vi "rad_Deploy Image Wrapper_FB.vi"(4 "Deploy":string[](array[string]), 6 "restart after imaging (T)":bool=TRUE, 7 "Deployment Notifiers":T3, 8 "error in (no error)":errorcluster, 9 "apply primary NIC from image (F)":bool, 10 "image file path":path, 11 "Target settings in":T1={"Hostname"="", "Serial number"="", "Product name"="", "Product code"=0, "System status"="", "Credential type"=enum."None/Unlocked", "User added?"=FALSE, "Primary NIC"={"MAC address"="", "IP Address Request Mode"=2, "IP address"="", "Subnet mask"="", "Gateway"="", "DNS server"=""}} {"Primary NIC"."IP Address Request Mode" items=["Static"=1, "DHCP/Link-Local"=2, "Link-Local Only"=4, "DHCP Only"=8]}) -> (0 "error out":errorcluster, 2 "image file path":path, 3 "Target settings out":T1={"Hostname"="", "Serial number"="", "Product name"="", "Product code"=0, "System status"="", "Credential type"=enum."None/Unlocked", "User added?"=FALSE, "Primary NIC"={"MAC address"="", "IP Address Request Mode"=2, "IP address"="", "Subnet mask"="", "Gateway"="", "DNS server"=""}} {"Primary NIC"."IP Address Request Mode" items=["Static"=1, "DHCP/Link-Local"=2, "Link-Local Only"=4, "DHCP Only"=8]})   [LabVIEW 2014]
uses:
  TypeDefs/rad_Deployment Notifiers.ctl
  TypeDefs/rad_Deployment Status Data Type.ctl
  TypeDefs/rad_Deployment Progress Data Type.ctl
  Targets/TypeDefs/rad_Target Information.ctl
  Targets/TypeDefs/rad_Target Network Settings.ctl
  <vilib>/nisyscfg/Network Settings Image.ctl
  <vilib>/nisyscfg/Set System Image (Folder).vi
  <vilib>/nisyscfg/Set System Image (File).vi
  <vilib>/nisyscfg/Close (System).vi
  <vilib>/nisyscfg/nisyscfg.lvlib
panel:
  out "finished":bool
  in  "Stop Checking for Events":bool
  out "Progress":u8(slide) scale=0.0..100.0
  out "Status":string
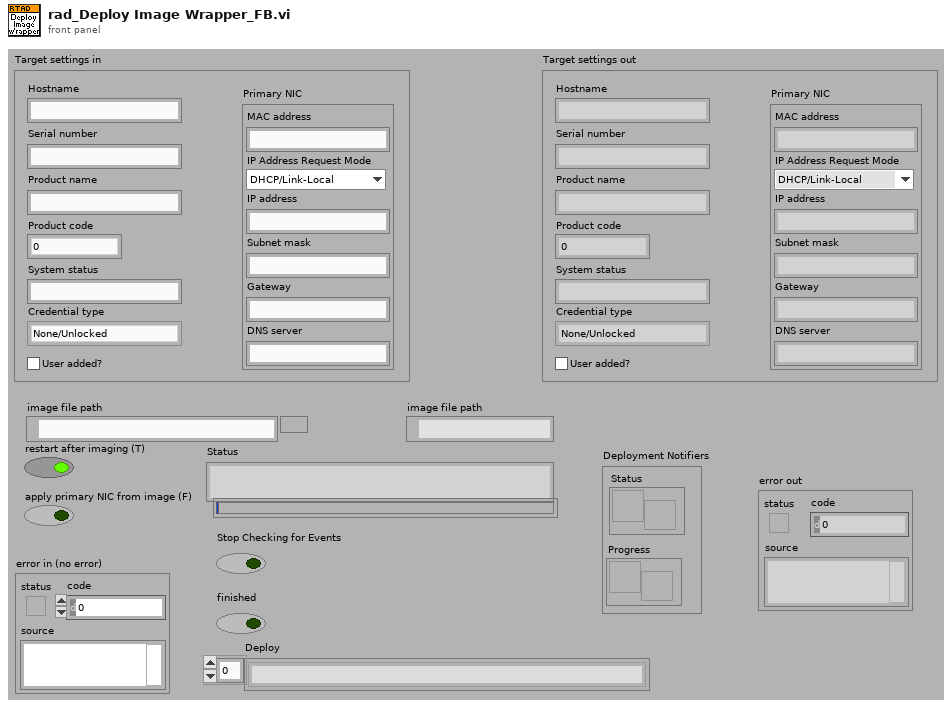
[diagram p1: front panel]
types:
  T1 = typedef "rad_Target Information.ctl" = cluster{"Hostname":string, "Serial number":string, "Product name":string, "Product code":i32, "System status":string, "Credential type":enum16{"None/Unlocked", "FTP Password", "NIAuth Credentials"}, "User added?":bool, "Primary NIC":T2}
  T2 = typedef "rad_Target Network Settings.ctl" = cluster{"MAC address":string, "IP Address Request Mode":i32, "IP address":string, "Subnet mask":string, "Gateway":string, "DNS server":string}
  T3 = typedef "rad_Deployment Notifiers.ctl" = cluster{"Status":refnum<notifier>, "Progress":refnum<notifier>}
  T4 = typedef "rad_Deployment Progress Data Type.ctl" = i8
  T5 = typedef "nisyscfg.lvlib/Network Settings Image.ctl" = u32
  T6 = enum32{"state changed", "beginning restart", "getting file", "putting file", "creating directory", "deleting file", "deleting directory", "enumerating file system", "renaming file", "current component", "operation progress", "downloading file", "unpacking file", "running install script"}
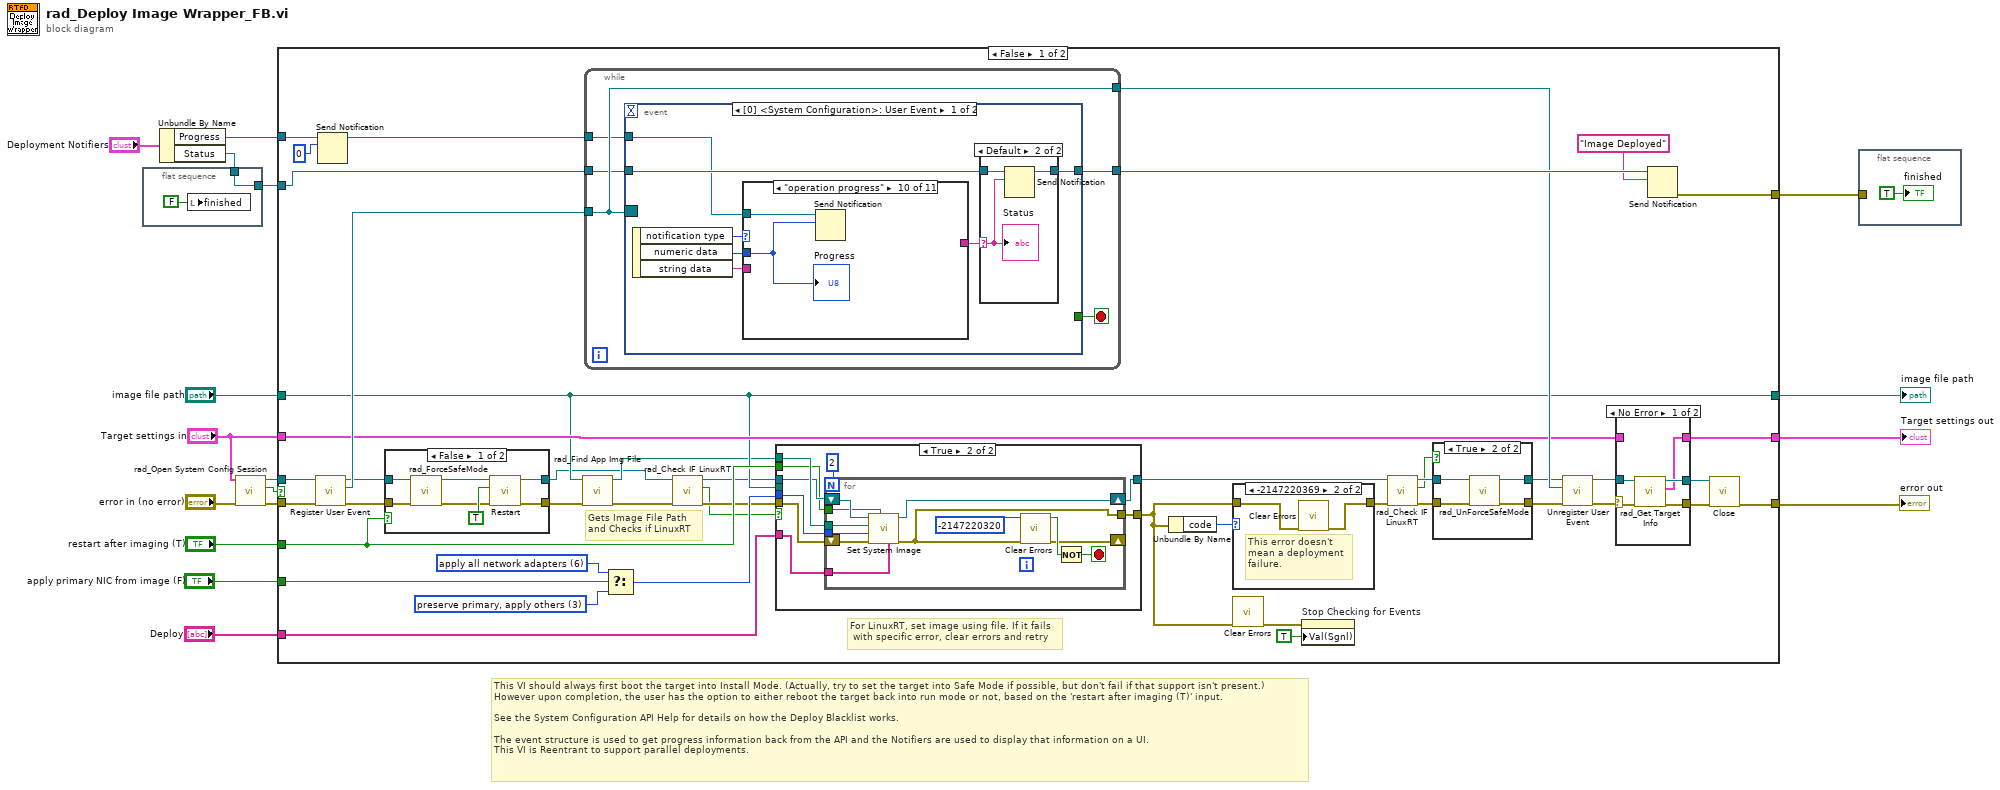
[diagram p0: block diagram]
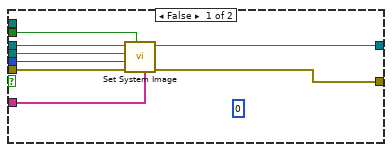
[diagram p2: hidden frame]
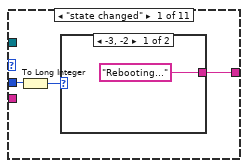
[diagram p8: hidden frame]
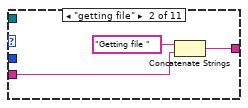
[diagram p10: hidden frame]
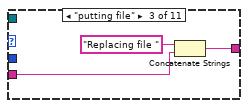
[diagram p11: hidden frame]
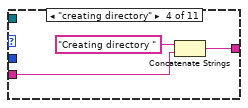
[diagram p12: hidden frame]
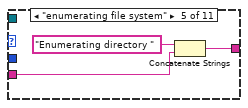
[diagram p13: hidden frame]
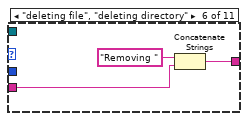
[diagram p14: hidden frame]
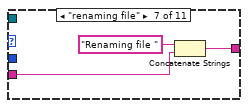
[diagram p15: hidden frame]
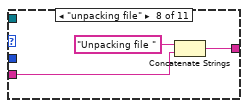
[diagram p16: hidden frame]
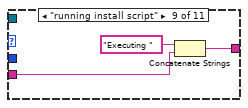
[diagram p17: hidden frame]
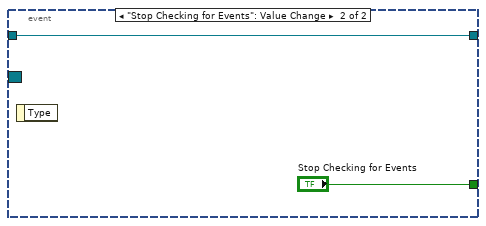
[diagram p19: hidden frame]
diagram:
  # "This VI should always first boot the target into Install Mode. (Actually, try to set the target into Safe Mode if possible, but don't fail if that support isn't present.)\nHowever upon completion, the user has the option to either reboot the target back into run mode or not, based on the 'restart after imaging (T)' input.\n\nSee the System Configuration API Help for details on how the Deploy Blacklist works.\n\nThe event structure is used to get progress information back from the API and the Notifiers are used to display that information on a UI. \nThis VI is Reentrant to support parallel deployments."
  n1 = flat-sequence {
    tunnel: [w18] -> w3
    tunnel: w2 -> [w18]
    frame #0 {
      n2 = local write "finished"(FALSE ("finished")) -> ()
    }
  }
  n3 = Unbundle By Name("Deployment Notifiers") -> ("Progress"=w11:refnum<notifier>, "Status"=w2:refnum<notifier>)
  n4 = call "rad_Open System Config Session.vi"("error in (no error)"="error in (no error)", "Target settings"="Target settings in") -> ("error out"=w7:errorcluster, "Cancelled"=w6:bool, "Session out"=w8:refnum<k21>)  [unwired: 6 in, 1 out]
  n5 = case shown="False" w6 {
    tunnel: [w64 w170] -> w17
    tunnel: "image file path" -> [w31 w169]
    tunnel: "restart after imaging (T)" -> [w47 _]
    tunnel: w8 -> [w63 _]
    tunnel: w7 -> [w62 w170]
    tunnel: [w58 _] -> w14
    tunnel: "apply primary NIC from image (F)" -> [w57 _]
    tunnel: w11 -> [w53 _]
    tunnel: [w31 w169] -> w16
    tunnel: "Deploy" -> [w33 _]
    tunnel: "Target settings in" -> [w34 w168]
    tunnel: [w44 w168] -> w4
    tunnel: w3 -> [w40 _]
    frame False {
      w56 = T5 6 items=["reset primary, disable others", "preserve primary, disable others", "preserve all network adapters", "preserve primary, apply others", "apply primary, disable others", "apply primary, preserve others", "apply all network adapters"] ("network settings (apply all adapters)")
      w55 = T5 3 items=["reset primary, disable others", "preserve primary, disable others", "preserve all network adapters", "preserve primary, apply others", "apply primary, disable others", "apply primary, preserve others", "apply all network adapters"] ("network settings (apply all adapters)")
      # "Gets Image File Path\nand Checks if LinuxRT"
      # "For LinuxRT, set image using file. If it fails\n with specific error, clear errors and retry"
      n6 = call <vilib>:"Register User Event.vi"("error in (no error)"=w62, "Session in"=w63) -> ("error out"=w48:errorcluster, "Event Registration out"=w61:refnum<event-registration>, "Session out"=w49:refnum<k21>)  [unwired: 7 in]
      n7 = Send Notification(notification=T4 0, notifier=w53) -> (notifier out=w52:refnum<notifier>)  [unwired: 1 in, 1 out]
      n8 = case shown="False" w47 {
        tunnel: w49 -> [w114 w116]
        tunnel: w48 -> [w109 w115]
        tunnel: [w112 w116] -> w28
        tunnel: [w111 w115] -> w32
        frame False {
          n9 = call "rad_ForceSafeMode.vi"("error in (no error)"=w109, "Target in"=w114) -> ("error out"=w108:errorcluster, "Target out"=w110:refnum<k21>)  [unwired: 8 in]
          n10 = call <vilib>:"Restart.vi"("error in (no error)"=w108, "Install Mode (F)"=TRUE ("install mode (F)"), "Session in"=w110) -> ("error out"=w111:errorcluster, "Session out"=w112:refnum<k21>)  [unwired: 6 in, 1 out]
        }
        frame True {
        }
      }
      n11 = call "rad_Find App Img File.vi"("Error In"=w32, "Temp Image Path"=w31) -> ("Error Out"=w29:errorcluster, "LVAppImg Path"=w30:path)  [unwired: 8 in]
      n12 = while {
        tunnel: w61 -> [w124]
        tunnel: [w124] -> w43
        tunnel: w40 -> [w122]
        tunnel: [w121] -> w60
        tunnel: w52 -> [w120]
        stop <- w123 stop-if-true
        n13 = event shown="[0] <System Configuration>: User Event" {
          selector: w124 -> [_ _]
          dyn-events: _ -> [_ _]
          timeout: _ -> [_ _]
          tunnel: [_ "Stop Checking for Events"] -> w123
          tunnel: w122 -> [w127 w166]
          tunnel: [w126 w166] -> w121
          tunnel: w120 -> [w125 _]
          event User Event {
            n14 = event-data() -> ("notification type"=w131:T6, "numeric data"=w129:u32, "string data"=w130:string)  [unwired: 1 in]
            n15 = case shown="\"operation progress\"" w131 {
              tunnel: [w136 w140 w143 w146 w149 w152 w155 w158 w161 _ _] -> w128
              tunnel: w130 -> [_ w141 w144 w147 w150 w153 w156 w159 w162 _ _]
              tunnel: w129 -> [w138 _ _ _ _ _ _ _ _ w165 _]
              tunnel: w125 -> [_ _ _ _ _ _ _ _ _ w164 _]
              frame "state changed" {
                n16 = To Long Integer(number=w138) -> (32bit integer=w137:i32)
                n17 = case shown="-3, -2" w137 {
                  tunnel: ["Rebooting..." _] -> w136
                  frame -3, -2 {
                  }
                  frame Default {
                  }
                }
              }
              frame "getting file" {
                n18 = Concatenate Strings("Getting file " ("Status"), w141) -> (w140:string)
              }
              frame "putting file" {
                n19 = Concatenate Strings("Replacing file " ("Status"), w144) -> (w143:string)
              }
              frame "creating directory" {
                n20 = Concatenate Strings("Creating directory " ("Status"), w147) -> (w146:string)
              }
              frame "enumerating file system" {
                n21 = Concatenate Strings("Enumerating directory " ("Status"), w150) -> (w149:string)
              }
              frame "deleting file", "deleting directory" {
                n22 = Concatenate Strings("Removing " ("Status"), w153) -> (w152:string)
              }
              frame "renaming file" {
                n23 = Concatenate Strings("Renaming file " ("Status"), w156) -> (w155:string)
              }
              frame "unpacking file" {
                n24 = Concatenate Strings("Unpacking file " ("Status"), w159) -> (w158:string)
              }
              frame "running install script" {
                n25 = Concatenate Strings("Executing " ("Status"), w162) -> (w161:string)
              }
              frame "operation progress" {
                n26 = Send Notification(notification=w165, notifier=w164) -> ()  [unwired: 1 in, 2 out]
                "Progress" <- w165
              }
              frame Default {
              }
            }
            n27 = case shown="Default" w128 {
              selector: w128 -> [_ w134]
              tunnel: w127 -> [w132 w135]
              tunnel: [w132 w133] -> w126
              frame "" {
              }
              frame Default {
                n28 = Send Notification(notification=w134, notifier=w135) -> (notifier out=w133:refnum<notifier>)  [unwired: 1 in, 1 out]
                "Status" <- w134
              }
            }
          }
          event "Stop Checking for Events": Value Change {
            n29 = event-data() -> ()  [unwired: 1 in, 1 out]
          }
        }
      }
      n30 = Select(t=w56, s=w57, f=w55) -> (s? t:f=w54:T5)
      n31 = call "rad_Check IF LinuxRT.vi"("Error In"=w29, "System Session In"=w28) -> ("Error Out"=w26:errorcluster, "Target is LinuxRT?"=w25:bool, "System Session Out"=w27:refnum<k21>)  [unwired: 5 in, 2 out]
      n32 = case shown="True" w25 {
        tunnel: w54 -> [w68 w78]
        tunnel: w31 -> [w69 _]
        tunnel: w27 -> [w70 w80]
        tunnel: w26 -> [w67 w77]
        tunnel: w47 -> [w71 w79]
        tunnel: [w65 w74] -> w38
        tunnel: [w72 w73] -> w22
        tunnel: w33 -> [w66 w75]
        tunnel: w30 -> [_ w81]
        frame False {
          (unwired) 0
          n33 = call-poly <vilib>:"Set System Image.vi"("File and Directory Blacklist"=w66, "Restart Automatically (T)"=w71, "error in (no error)"=w67, "Network Settings (preserve primary adapter, apply others)"=w68, "Source Folder"=w69, "Session in"=w70) -> ("error out"=w65:errorcluster, "Session out"=w72:refnum<k21>)  [unwired: 4 in]
        }
        frame True {
          n34 = for {
            N: 2 -> [_]
            tunnel: w81 -> [w93]
            tunnel: w79 -> [w91]
            tunnel: w78 -> [w90]
            tunnel: w75 -> [w88]
            tunnel: [w83] -> w74
            shift-right: [w85] -> _
            shift-left: w77 -> [w89]
            shift-right: [w84] -> w73
            shift-left: w80 -> [w92]
            stop <- w87 stop-if-true
            n35 = call-poly <vilib>:"Set System Image.vi"("File and Directory Blacklist"=w88, "Restart Automatically (T)"=w91, "error in (no error)"=w89, "Network Settings (preserve primary adapter, apply others)"=w90, "Source File"=w93, "Session in"=w92) -> ("error out"=w83:errorcluster, "Session out"=w84:refnum<k21>)  [unwired: 4 in]
            n36 = call <vilib>:"Clear Errors.vi"("error in (no error)"=w83, "specific error code to clear (0: all)"=-2147220320) -> ("error out"=w85:errorcluster, "specific error cleared?"=w86:bool)  [unwired: 4 in]
            n37 = Not(x=w86) -> (.not. x?=w87:bool)
          }
        }
      }
      n38 = Unbundle By Name(w38) -> ("code"=w50:i32)
      n39 = case shown="-2147220369" w50 {
        tunnel: w38 -> [w117 w119]
        tunnel: [w117 w118] -> w24
        frame Default {
        }
        frame -2147220369 {
          # "This error doesn't\nmean a deployment\nfailure."
          n40 = call <vilib>:"Clear Errors.vi"("error in (no error)"=w119) -> ("error out"=w118:errorcluster)  [unwired: 5 in, 1 out]
        }
      }
      n41 = call <vilib>:"Clear Errors.vi"("error in (no error)"=w38) -> ("error out"=w37:errorcluster)  [unwired: 5 in, 1 out]
      n42 = property on="Stop Checking for Events" class="Bool (strict)"(error in=w37, "Val(Sgnl)"=TRUE ("Stop Checking for Events")) -> ()  [unwired: 1 in, 2 out]
      n43 = call "rad_Check IF LinuxRT.vi"("Error In"=w24, "System Session In"=w22) -> ("Error Out"=w23:errorcluster, "Target is LinuxRT?"=w20:bool, "System Session Out"=w21:refnum<k21>)  [unwired: 5 in, 2 out]
      n44 = case shown="True" w20 {
        tunnel: w21 -> [w95 w99]
        tunnel: w23 -> [w94 w98]
        tunnel: [w94 w96] -> w36
        tunnel: [w95 w97] -> w35
        frame False {
        }
        frame True {
          n45 = call "rad_UnForceSafeMode.vi"("error in (no error)"=w98, "Target in"=w99) -> ("error out"=w96:errorcluster, "Target out"=w97:refnum<k21>)  [unwired: 8 in]
        }
      }
      n46 = call <vilib>:"Unregister User Event.vi"("error in (no error)"=w36, "Event Registration in"=w43, "Session in"=w35) -> ("error out"=w42:errorcluster, "Session out"=w41:refnum<k21>)  [unwired: 7 in]
      n47 = case shown="No Error" w42 {
        selector: w42 -> [w103 w107]
        tunnel: [w101 w107] -> w46
        tunnel: w41 -> [w104 w106]
        tunnel: [w102 w106] -> w45
        tunnel: [w100 w105] -> w44
        tunnel: w34 -> [_ w105]
        frame No Error {
          n48 = call "rad_Get Target Info.vi"("error in (no error)"=w103, "System Session in"=w104) -> ("error out"=w101:errorcluster, "Target settings"=w100:T1, "System Session out"=w102:refnum<k21>)  [unwired: 7 in]
        }
        frame Error {
        }
      }
      n49 = Send Notification(notification="Image Deployed", notifier=w60) -> (error out=w58:errorcluster)  [unwired: 1 in, 1 out]
      n50 = call-poly <vilib>:"Close.vi"("error in (no error)"=w46, "Session in"=w45) -> ("error out"=w64:errorcluster)  [unwired: 9 in]
    }
    frame True {
    }
  }
  "error out" <- w17
  "image file path" <- w16
  "Target settings out" <- w4
  n51 = flat-sequence {
    tunnel: w14 -> [_]
    frame #0 {
      "finished" <- TRUE ("finished")
    }
  }
